vi "15-Extra.vi"() -> ()   [LabVIEW 2019, in "15.lvlib"]
uses:
  15.lvlib
panel:
  in  "Duplicate?":bool
  out "Risk Relief":u8[][](graph)
  out "Min Path Risk Relief":i32[][](graph)
  in  "Sample Input?":bool
  out "Min Risk":u64
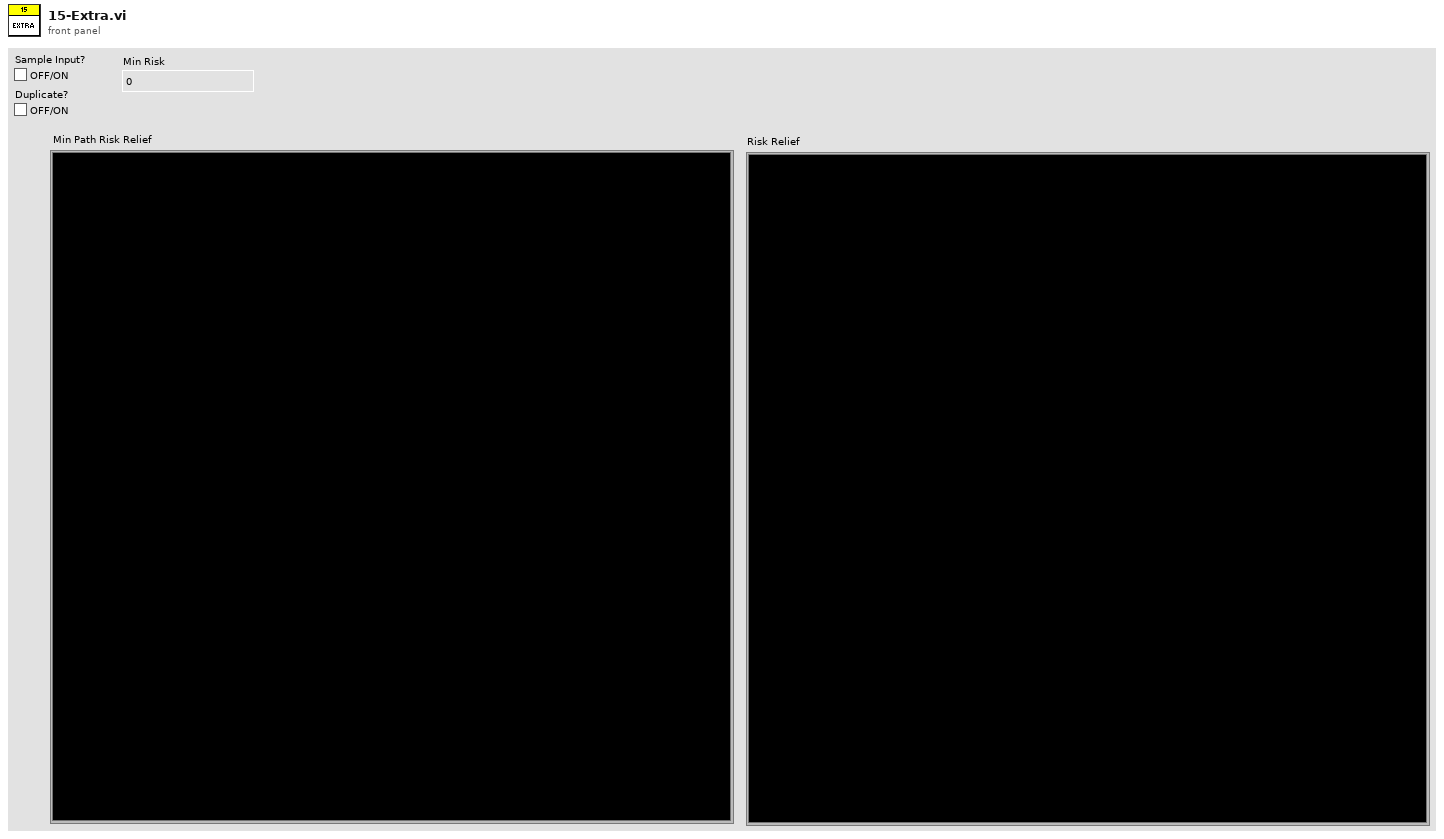
[diagram p1: front panel]
types:
  T1 = map{cluster{"Row":i32, "Col":i32}, cluster{"Adjacency Matrix":cluster{i32, i32}[], "Risk":u8, "Min Risk":i32, "Visited?":bool}}
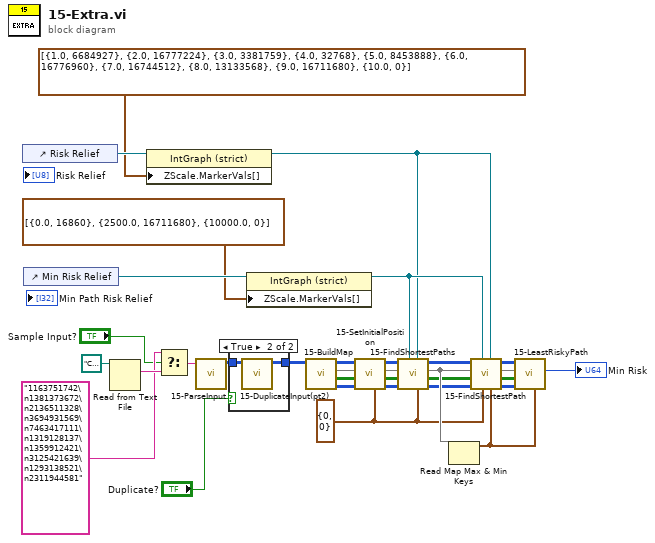
[diagram p0: block diagram]
diagram:
  w10 = cluster{"Row":i32, "Col":i32} {"Row"=0, "Col"=0} ("Initial Position in")
  n1 = control-ref of="Risk Relief"() -> (w19:refnum<vi>)
  n2 = control-ref of="Min Risk Relief"() -> (w21:refnum<vi>)
  n3 = Read from Text File(file (use dialog)=path "C:/Users/craig.walker/Documents/GitHub/lv2019-Advent-of-Code-2021/15/input.txt") -> (text=w28:string)  [unwired: 3 in, 3 out]
  n4 = property class="IntGraph (strict)"(reference=w19, "ZScale.MarkerVals[]"=cluster{dbl, u32}[] [{1.0, 6684927}, {2.0, 16777224}, {3.0, 3381759}, {4.0, 32768}, {5.0, 8453888}, {6.0, 16776960}, {7.0, 16744512}, {8.0, 13133568}, {9.0, 16711680}, {10.0, 0}] ("Z Scale.Marker Values[]")) -> (reference out=w5:refnum<vi>)  [unwired: 1 in, 1 out]
  n5 = Select(t="1163751742\n1381373672\n2136511328\n3694931569\n7463417111\n1319128137\n1359912421\n3125421639\n1293138521\n2311944581", s="Sample Input?", f=w28) -> (s? t:f=w29:string)
  n6 = call "15-ParseInput.vi"("String"=w29) -> ("Risk Array"=w30:u8[][])  [unwired: 10 in]
  n7 = case shown="True" "Duplicate?" {
    tunnel: w30 -> [w34 w36]
    tunnel: [w34 w35] -> w17
    frame False {
    }
    frame True {
      n8 = call "15-DuplicateInput(pt2).vi"("Risk Array in"=w36) -> ("Risk Array out"=w35:u8[][])  [unwired: 10 in]
    }
  }
  n9 = property class="IntGraph (strict)"(reference=w21, "ZScale.MarkerVals[]"=cluster{dbl, u32}[] [{0.0, 16860}, {2500.0, 16711680}, {10000.0, 0}] ("Z Scale.Marker Values[]")) -> (reference out=w7:refnum<vi>)  [unwired: 1 in, 1 out]
  n10 = call "15-BuildMap.vi"("Risk Array in"=w17) -> ("Min Risk Array"=w15:i32[][], "Visited Array"=w23:bool[][], "map"=w31:T1, "Risk Array out"=w16:u8[][])  [unwired: 7 in]
  n11 = call "15-SetInitialPosition.vi"("Initial Position in"=w10, "Min Risk Array in"=w15, "Visited Array in"=w23, "map in"=w31, "Risk Array in"=w16) -> ("Min Risk Array out"=w14:i32[][], "Visited Array out"=w22:bool[][], "map out"=w25:T1, "Risk Array out"=w32:u8[][])  [unwired: 3 in]
  n12 = call "15-FindShortestPaths.vi"("Risk Relief"=w5, "Initial Position in"=w10, "Min Risk Relief"=w7, "Min Risk Array in"=w14, "Visited Array in"=w22, "map in"=w25, "Risk Array in"=w32) -> ("Min Risk Array out"=w9:i32[][], "Visited Array out"=w6:bool[][], "map out"=w13:T1, "Risk Array out"=w8:u8[][])  [unwired: 1 in]
  n13 = Read Map Max & Min Keys(11:w13) -> (3:w11:cluster{"Row":i32, "Col":i32})  [unwired: 1 out]
  n14 = call "15-FindShortestPath.vi"("Final Position"=w11, "Risk Relief"=w5, "Initial Position"=w10, "Min Path Risk Relief"=w7, "Min Risk Array in"=w9, "Visited Array in"=w6, "map in"=w13, "Risk Array in"=w8) -> ("Min Risk Array out"=w2:i32[][], "Visited Array out"=w3:bool[][], "map out"=w12:T1, "Risk Array out"=w4:u8[][])
  n15 = call "15-LeastRiskyPath.vi"("Final Position"=w11, "Min Risk Array in"=w2, "Visited Array in"=w3, "map in"=w12, "Risk Array in"=w4) -> ("Min Risk"=→"Min Risk":i32)  [unwired: 3 in, 3 out]
